vi "AutoCentral.vi"(3 "ConfigurationFile":path=path "E:/Code/Tasks/FingerMove/FingerMove_CerebusConfig.ccf", 5 "Mode":T1(ring)) -> (0 "Path":path=path "E:/Code/PID/SubVIs", 1 "DataFolder":string, 2 "Recording?":bool)   [LabVIEW 2012]
panel:
  out "Result":string="Initializing Cerebus real-time interface 6.03.00.00 (protocol cb3.08)...\r\nCentral real-time interface to NSP (6.03.00.00) successfully initialized\r\nInterface closed successfully\r\nRecording stopped successfully\r\n"
  in  "ExecutableFile":path=path "E:/Code/Tasks/TaskAutomation/autoCentral.exe"
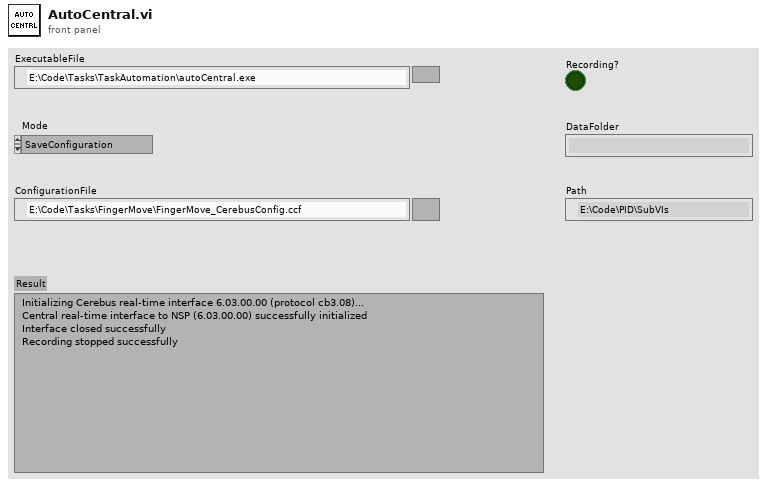
[diagram p1: front panel]
types:
  T1 = enum16{"SaveConfiguration", "StartRecording", "StopRecording"}
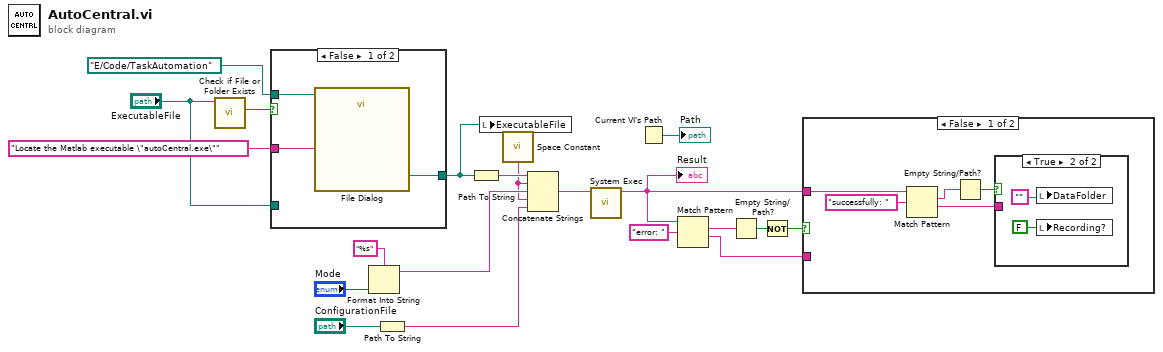
[diagram p0: block diagram]
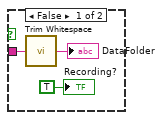
[diagram p3: hidden frame]
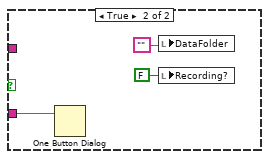
[diagram p4: hidden frame]
diagram:
  n1 = call <vilib>:"Check if File or Folder Exists.vi"("path"="ExecutableFile") -> ("file or folder exists?"=w9:bool)  [unwired: 8 in, 2 out]
  n2 = case shown="False" w9 {
    tunnel: "ExecutableFile" -> [_ w24]
    tunnel: [w23 w24] -> w7
    tunnel: "Locate the Matlab executable \"autoCentral.exe\"" -> [w22 _]
    tunnel: path "E:/Code/TaskAutomation" -> [w21 _]
    frame False {
      n3 = call "File Dialog"("start path"=w21, "prompt"=w22) -> ("selected path"=w23:path)  [unwired: 10 in, 3 out]
    }
    frame True {
    }
  }
  n4 = Format Into String(format string="%s", "Mode") -> (resulting string=w14:string)  [unwired: 2 in, 1 out]
  n5 = Path To String(path="ConfigurationFile") -> (string=w4:string)
  n6 = Path To String(path=w7) -> (string=w12:string)
  n7 = local write "ExecutableFile"(w7) -> ()
  n8 = call <vilib>:"Space Constant.vi"() -> ("String"=w11:string)
  n9 = Concatenate Strings(w12, w11, w14, w11, w4) -> (w10:string)
  n10 = call <vilib>:"System Exec.vi"("command line"=w10) -> ("standard output"=w2:string)  [unwired: 7 in, 3 out]
  "Result" <- w2
  n11 = Current VI's Path() -> (path=→"Path":path)
  n12 = Match Pattern(string=w2, regular expression="error: ") -> (match substring=w19:string, after substring=w16:string)  [unwired: 1 in, 2 out]
  n13 = Empty String/Path?(string/path=w19) -> (empty?=w18:bool)
  n14 = Not(x=w18) -> (.not. x?=w17:bool)
  n15 = case shown="False" w17 {
    tunnel: w16 -> [_ w37]
    tunnel: w2 -> [w28 _]
    frame False {
      n16 = Match Pattern(string=w28, regular expression="successfully: ") -> (match substring=w26:string, after substring=w27:string)  [unwired: 1 in, 2 out]
      n17 = Empty String/Path?(string/path=w26) -> (empty?=w25:bool)
      n18 = case shown="True" w25 {
        tunnel: w27 -> [w32 _]
        frame False {
          n19 = call <vilib>:"Trim Whitespace.vi"("string"=w32) -> ("trimmed string"=→"DataFolder":string)  [unwired: 1 in]
          "Recording?" <- TRUE
        }
        frame True {
          n20 = local write "DataFolder"("") -> ()
          n21 = local write "Recording?"(FALSE ("Recording?")) -> ()
        }
      }
    }
    frame True {
      n22 = One Button Dialog(message=w37) -> ()  [unwired: 1 in, 1 out]
      n23 = local write "DataFolder"("") -> ()
      n24 = local write "Recording?"(FALSE ("Recording?")) -> ()
    }
  }
